vi "send_Sensorbox.vi"(4 "Counter":i32, 5 "200/freq":i32=1, 6 "Active":bool, 7 "CAN ID":u32[](array[numeric])=[372, 376, 380] format="%x", 8 "Message":T2 {"Roll [°/s]" scale=-150.0..150.0; "Yaw [°/s]" scale=-150.0..150.0; "Acc Z [g]" scale=-4.1..4.1; "Acc Y [g]" scale=-4.1..4.1; "Acc X [g]" scale=-4.1..4.1}, 11 "CAN frame":T1[](array[typedef]) {"Data" format="%.0x"; "ArbitrationId" format="%.0x"; "Timestamp" format="%<%I:%M:%S%3u %p\n%m/%d/%Y>T"}) -> (3 "CAN frame out":T1[](array[typedef]) {"Data" format="%.0x"; "ArbitrationId" format="%.0x"; "Timestamp" format="%<%I:%M:%S%3u %p\n%m/%d/%Y>T"})   [LabVIEW 2017]
uses:
  <vilib>/nican/nican.llb/CanFrameTimed.ctl
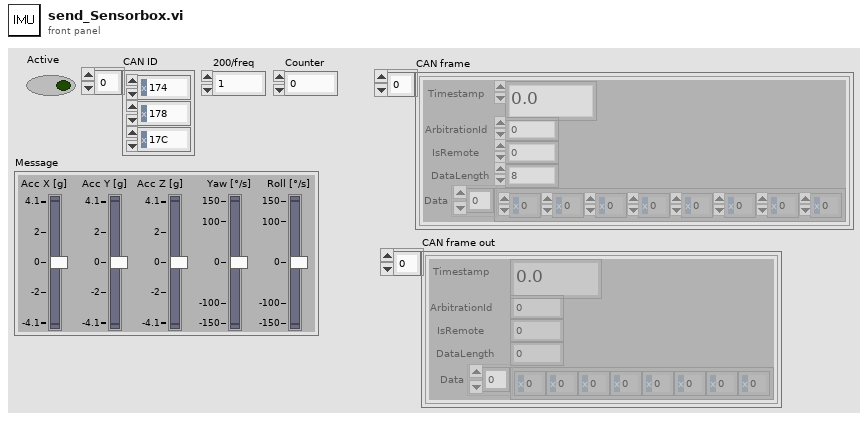
[diagram p1: front panel]
types:
  T1 = typedef "CanFrameTimed.ctl" = cluster{"Timestamp":dbl, "ArbitrationId":u32, "IsRemote":u8, "DataLength":u8, "Data":u8[]}
  T2 = cluster{"Acc X [g]":dbl, "Acc Y [g]":dbl, "Acc Z [g]":dbl, "Yaw [°/s]":dbl, "Roll [°/s]":dbl}
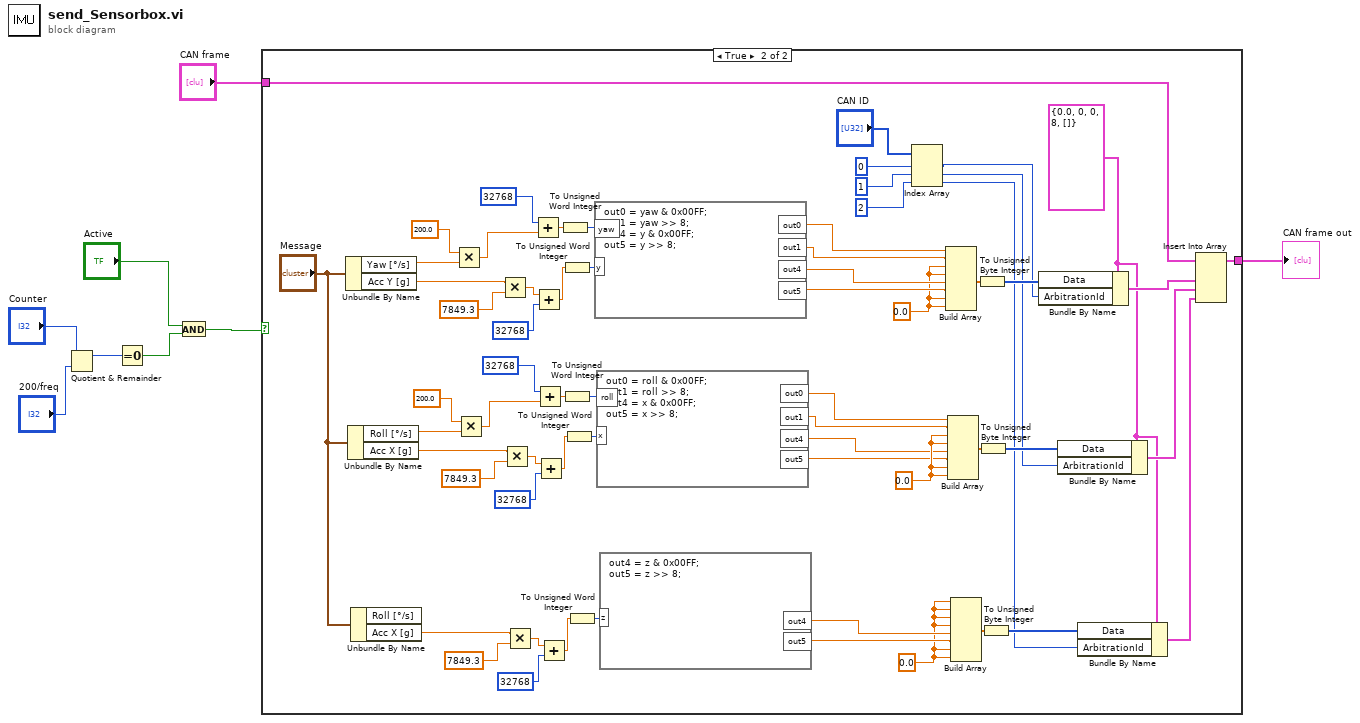
[diagram p0: block diagram]
diagram:
  n1 = Quotient & Remainder(x="Counter", y="200/freq") -> (x-y*floor(x/y)=w5:i32)  [unwired: 1 out]
  n2 = Equal To 0?(x=w5) -> (x = 0?=w3:bool)
  n3 = And(x="Active", y=w3) -> (x .and. y?=w2:bool)
  n4 = case shown="True" w2 {
    tunnel: "CAN frame" -> [w9 w68]
    tunnel: [w9 w66] -> w7
    frame False {
    }
    frame True {
      w14 = 0.0 ("element")
      w45 = 0.0 ("element")
      w46 = 0.0 ("element")
      w13 = T1 {"Timestamp"=0.0, "ArbitrationId"=0, "IsRemote"=0, "DataLength"=8, "Data"=[]} ("CAN frame")
      n5 = Unbundle By Name("Message") -> ("Yaw [°/s]"=w65:dbl, "Acc Y [g]"=w53:dbl)
      n6 = Unbundle By Name("Message") -> ("Roll [°/s]"=w31:dbl, "Acc X [g]"=w38:dbl)
      n7 = Unbundle By Name("Message") -> ("Acc X [g]"=w21:dbl)  [unwired: 1 out]
      n8 = Multiply(x=200.0, y=w65) -> (x*y=w54:dbl)
      n9 = Multiply(x=200.0, y=w31) -> (x*y=w37:dbl)
      n10 = Multiply(x=w53, y=7849.3 ("x")) -> (x*y=w51:dbl)
      n11 = Multiply(x=w38, y=7849.3 ("x")) -> (x*y=w40:dbl)
      n12 = Multiply(x=w21, y=7849.3 ("x")) -> (x*y=w19:dbl)
      n13 = Add(x=u16 32768, y=w54) -> (x+y=w55:dbl)
      n14 = Add(x=w51, y=u16 32768 ("x")) -> (x+y=w49:dbl)
      n15 = Add(x=u16 32768, y=w37) -> (x+y=w36:dbl)
      n16 = Add(x=w40, y=u16 32768 ("x")) -> (x+y=w42:dbl)
      n17 = Add(x=w19, y=u16 32768 ("x")) -> (x+y=w17:dbl)
      n18 = To Unsigned Word Integer(number=w55) -> (unsigned 16bit integer=w56:u16)
      n19 = To Unsigned Word Integer(number=w49) -> (unsigned 16bit integer=w72:u16)
      n20 = To Unsigned Word Integer(number=w36) -> (unsigned 16bit integer=w35:u16)
      n21 = To Unsigned Word Integer(number=w42) -> (unsigned 16bit integer=w27:u16)
      n22 = To Unsigned Word Integer(number=w17) -> (unsigned 16bit integer=w24:u16)
      n23 = formula code="out0 = yaw & 0x00FF;\nout1 = yaw >> 8;\nout4 = y & 0x00FF;\nout5 = y >> 8;"("y"=w72, "yaw"=w56) -> ("out1"=w71:dbl, "out4"=w47:dbl, "out5"=w48:dbl, "out0"=w63:dbl)
      n24 = formula code="out0 = roll & 0x00FF;\nout1 = roll >> 8;\nout4 = x & 0x00FF;\nout5 = x >> 8;"("x"=w27, "roll"=w35) -> ("out1"=w28:dbl, "out4"=w44:dbl, "out5"=w43:dbl, "out0"=w33:dbl)
      n25 = formula code="out4 = z & 0x00FF;\nout5 = z >> 8;"("z"=w24) -> ("out4"=w15:dbl, "out5"=w16:dbl)
      n26 = Index Array(array="CAN ID", index #1=0 ("index"), index #2=1 ("index"), index #3=2 ("index")) -> (element #1=w61:u32, element #2=w26:u32, element #3=w11:u32)
      n27 = Build Array(w63, w71, w46, w46, w47, w48, w46, w46) -> (w70:dbl[])
      n28 = Build Array(w33, w28, w45, w45, w44, w43, w45, w45) -> (w29:dbl[])
      n29 = Build Array(w14, w14, w14, w14, w15, w16, w14, w14) -> (w23:dbl[])
      n30 = To Unsigned Byte Integer(number=w70) -> (unsigned 8bit integer=w69:u8[])
      n31 = To Unsigned Byte Integer(number=w29) -> (unsigned 8bit integer=w30:u8[])
      n32 = To Unsigned Byte Integer(number=w23) -> (unsigned 8bit integer=w22:u8[])
      n33 = Bundle By Name(cluster=w13, "Data"=w69, "ArbitrationId"=w61) -> (w67:T1)
      n34 = Bundle By Name(cluster=w13, "Data"=w30, "ArbitrationId"=w26) -> (w25:T1)
      n35 = Bundle By Name(cluster=w13, "Data"=w22, "ArbitrationId"=w11) -> (w12:T1)
      n36 = Insert Into Array(array=w68, new element #1=w67, new element #2=w25, new element #3=w12) -> (w66:T1[])  [unwired: 1 in]
    }
  }
  "CAN frame out" <- w7
